vi "test Empty Executable Name.vi"(8 "error in":errorcluster) -> (0 "error out":errorcluster)   [LabVIEW 2020, in "ase.test.lvlib"]
uses:
  ase.test.lvlib
  ase/ase/ase.lvclass/ase.ctl
  ase/ase/Trim Whitespace.vi
  ase/ase/Check Shared Library Version.vi
  ase/ase/Merge Call Library Errors.vi
  ase/ase/Error Invalid ASE Handle.vi
  ase/ase/Error Internal Library Implementation Error.vi
  <vilib>/Utility/error.llb/Error Cluster From Error Code.vi
  ase/ase/Wait on Call.vi
  <vilib>/addons/_JKI Toolkits/Caraya/classes/Assert/Assert Equal Value and Type_Variant.vi
  ase/ase/ase.lvclass
  <vilib>/addons/_JKI Toolkits/Caraya/classes/Assert/Assert.lvclass
  <vilib>/addons/_JKI Toolkits/Caraya/classes/Test/Test.lvclass
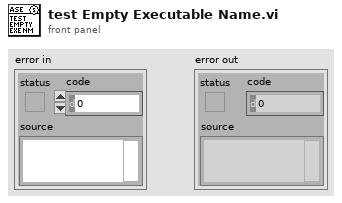
[diagram p1: front panel]
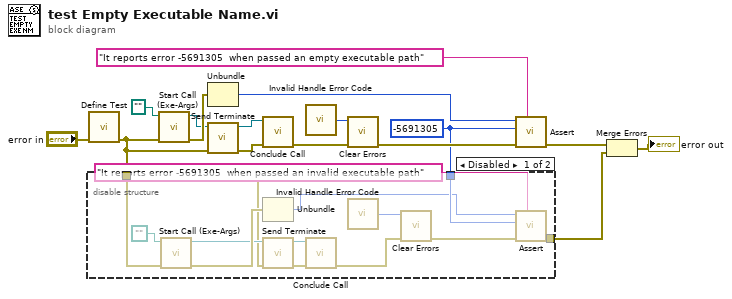
[diagram p0: block diagram]
diagram:
  w1 = -5691305 ("error code (1)")
  n1 = call <vilib>:"Define Test.vi"("error in (no error)"="error in") -> ("error out"=w3:errorcluster)  [unwired: 9 in, 1 out]
  n2 = disable-structure shown="Disabled" {
    disable-tunnel: w3 -> [w21 _]
    disable-tunnel: [w20 _] -> w2
    disable-tunnel: w1 -> [w19 _]
    frame Disabled {
      n3 = call "Start Call (Exe-Args).vi"("error in"=w21, "Executable Path"=path "") -> ("error out"=w25:errorcluster, "New ASE Handle"=w22:refnum<class "ase.lvclass">)  [unwired: 8 in]
      n4 = Unbundle(w25) -> ("code"=w18:i32)  [unwired: 2 out]
      n5 = call "Send Terminate.vi"("error in"=w21, "ASE Handle"=w22) -> ("error out"=w24:errorcluster, "ASE Handle Duplicate"=w26:refnum<class "ase.lvclass">)  [unwired: 7 in, 1 out]
      n6 = call "Conclude Call.vi"("error in"=w24, "ASE Handle"=w26) -> ("error out"=w28:errorcluster)  [unwired: 7 in, 2 out]
      n7 = call "Invalid Handle Error Code.vi"() -> ("Invalid Handle Error"=w27:i32)
      n8 = call <vilib>:"Clear Errors.vi"("error in (no error)"=w28, "specific error code to clear (0: all)"=w27) -> ("error out"=w29:errorcluster)  [unwired: 4 in, 1 out]
      n9 = call-poly <vilib>:"Assert.vi"("Label"="It reports error -5691305  when passed an invalid executable path", "error in (no error)"=w29, "Y"=w19, "X"=w18) -> ("error out"=w20:errorcluster)  [unwired: 6 in, 1 out]
    }
    frame Enabled {
    }
  }
  n10 = call "Start Call (Exe-Args).vi"("error in"=w3, "Executable Path"=path "") -> ("error out"=w14:errorcluster, "New ASE Handle"=w10:refnum<class "ase.lvclass">)  [unwired: 8 in]
  n11 = Unbundle(w14) -> ("code"=w5:i32)  [unwired: 2 out]
  n12 = call "Send Terminate.vi"("error in"=w3, "ASE Handle"=w10) -> ("error out"=w15:errorcluster, "ASE Handle Duplicate"=w13:refnum<class "ase.lvclass">)  [unwired: 7 in, 1 out]
  n13 = call "Conclude Call.vi"("error in"=w15, "ASE Handle"=w13) -> ("error out"=w11:errorcluster)  [unwired: 7 in, 2 out]
  n14 = call "Invalid Handle Error Code.vi"() -> ("Invalid Handle Error"=w12:i32)
  n15 = call <vilib>:"Clear Errors.vi"("error in (no error)"=w11, "specific error code to clear (0: all)"=w12) -> ("error out"=w8:errorcluster)  [unwired: 4 in, 1 out]
  n16 = call-poly <vilib>:"Assert.vi"("Label"="It reports error -5691305  when passed an empty executable path", "error in (no error)"=w8, "Y"=w1, "X"=w5) -> ("error out"=w6:errorcluster)  [unwired: 6 in, 1 out]
  n17 = Merge Errors(w6, w2) -> (→"error out":errorcluster)
